vi "Create User Event.vi"(8 "Error In":errorcluster) -> (0 "Error Out":errorcluster)   [LabVIEW 2017]
uses:
  Reference Action.ctl
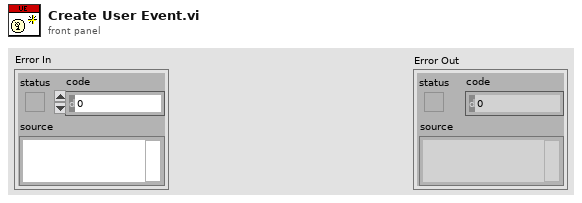
[diagram p1: front panel]
types:
  T1 = typedef "Reference Action.ctl" = enum16{"Set", "Get"}
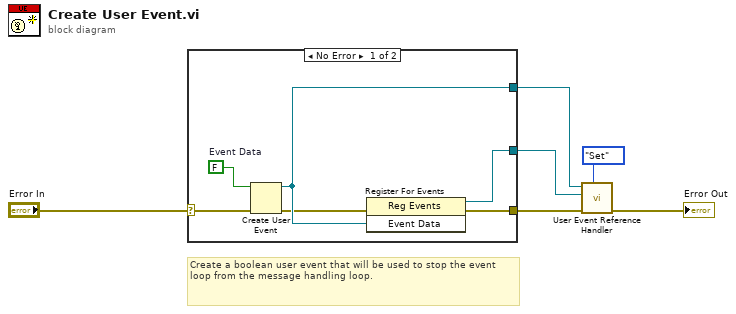
[diagram p0: block diagram]
diagram:
  # "Create a boolean user event that will be used to stop the event loop from the message handling loop."
  n1 = case shown="No Error" "Error In" {
    selector: "Error In" -> [w7 w13]
    tunnel: [w12 _] -> w5
    tunnel: [w11 _] -> w4
    tunnel: [w8 w13] -> w3
    frame No Error {
      w10 = FALSE  # Event Data
      n2 = Create User Event(user event datatype=w10, error in=w7) -> (user event=w12:refnum<user-event>, error out=w9:errorcluster)
      n3 = register-events(error in=w9, w12) -> (reference out=w11:refnum<event-registration>, error out=w8:errorcluster)  [unwired: 1 in]
    }
    frame Error {
    }
  }
  n4 = call "User Event Reference Handler.vi"("Reference Action"=Reference_Action."Set", "Error In"=w3, "Event Registration Refnum In"=w4, "User Event Refnum In"=w5) -> ("Error Out"=→"Error Out":errorcluster)  [unwired: 5 in, 2 out]
